vi "Format Voltage.vi"(8 "error in (no error)":errorcluster, 10 "String In":string, 11 "Fluke Calibrator in":refnum<class "Fluke Calibrator.lvclass">) -> (0 "error out":errorcluster, 2 "Number out":dbl, 3 "Fluke Calibrator out":refnum<class "Fluke Calibrator.lvclass">)   [LabVIEW 2012, in "Fluke Calibrator.lvclass"]
uses:
  Fluke Calibrator.lvclass
  Fluke Calibrator.lvclass/Fluke Calibrator.ctl
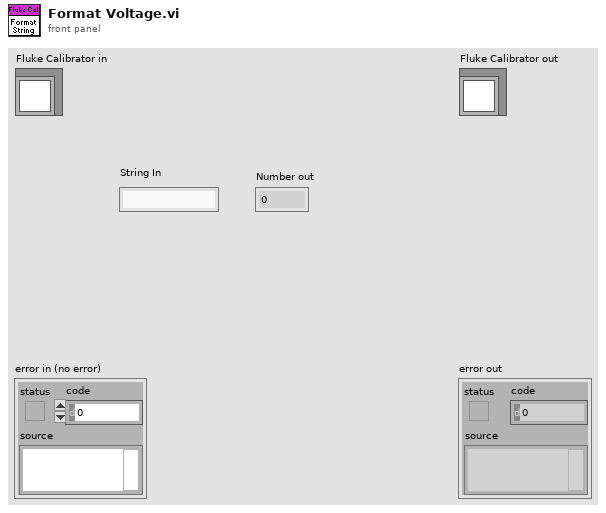
[diagram p1: front panel]
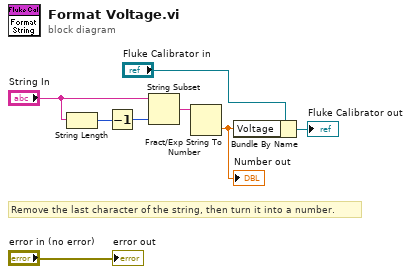
[diagram p0: block diagram]
diagram:
  # "Remove the last character of the string, then turn it into a number."
  n1 = String Length(string="String In") -> (length=w8:i32)
  n2 = Decrement(x=w8) -> (x-1=w7:i32)
  n3 = String Subset(string="String In", length (rest)=w7) -> (substring=w6:string)  [unwired: 1 in]
  n4 = Fract/Exp String To Number(string=w6) -> (number=w1:dbl)  [unwired: 3 in, 1 out]
  "Number out" <- w1
  n5 = Bundle By Name(cluster="Fluke Calibrator in", "Voltage"=w1) -> (→"Fluke Calibrator out":refnum<class "Fluke Calibrator.lvclass">)
  "error out" <- "error in (no error)"
